vi "In Series_.vi"(7 "Tolerance (%)":dbl, 8 "error in (no error)":errorcluster, 9 "Number of Bands":T1=4 min=3 max=6 step=1, 10 "Resistance Digits":T2, 11 "E-Series Data":T5) -> (0 "error out":errorcluster, 3 "In Series?":T4)   [LabVIEW 2018]
doc: "Determines the E-Series membership of a resistor based on its number of bands, tolerance, and significant digits.\n\nThe VI receives the <b>E-Series Data</b>, <b>Tolerance (%)</b>, <b>Number of Bands</b>, and <b>Resistance Digits</b>. It uses <b>Build Resistor Cipher.vi</b> to construct the resistance value represented by the selected digits.\n\nBased on the number of bands and the resistor tolerance, the VI evaluates the applicable E-Series values and determines which series contain the resistance value.\n\nThe result is returned through <b>In Series?</b>, a cluster of Boolean indicators corresponding to E3, E6, E12, E24, E48, E96, and E192.\n\nThe VI propagates errors through its <b>error in</b> and <b>error out</b> terminals."
uses:
  E-Series Reader/Series Data--cluster.ctl
  In series--cluster.ctl
  Resistance Digits--cluster.ctl
  Ddigit--enum.ctl
  Number of Bands--number.ctl
  Resistance Value/Resistance Value.lvlib
  E-Series Reader/E-Series Reader.lvlib
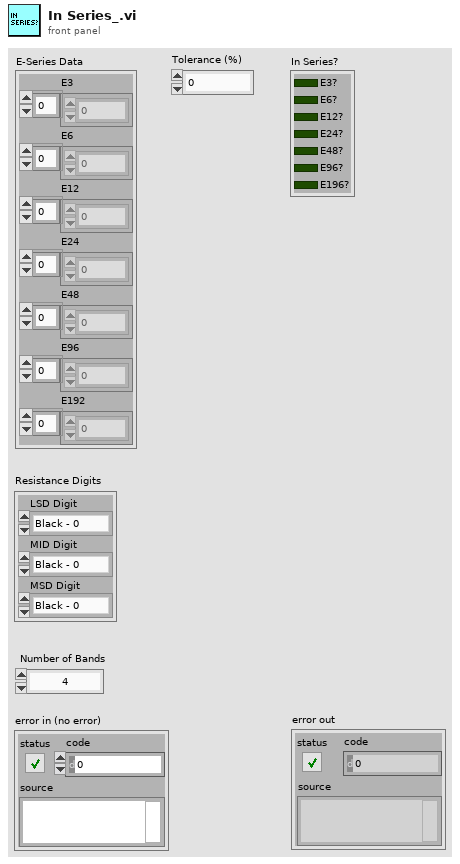
[diagram p1: front panel]
types:
  T1 = typedef "Number of Bands--number.ctl" = u8
  T2 = typedef "Resistance Digits--cluster.ctl" = cluster{"LSD Digit":T3, "MID Digit":T3, "MSD Digit":T3}
  T3 = typedef "Ddigit--enum.ctl" = enum16{"Black - 0", "Brown - 1", "Red - 2", "Orange - 3", "Yellow - 4", "Green - 5", "Blue - 6", "Violet - 7", "Grey - 8", "White - 9"}
  T4 = typedef "In series--cluster.ctl" = cluster{"E3?":bool, "E6?":bool, "E12?":bool, "E24?":bool, "E48?":bool, "E96?":bool, "E196?":bool}
  T5 = typedef "E-Series Reader.lvlib/Series Data--cluster.ctl" = cluster{"E3":u16[], "E6":u16[], "E12":u16[], "E24":u16[], "E48":u16[], "E96":u16[], "E192":u16[]}
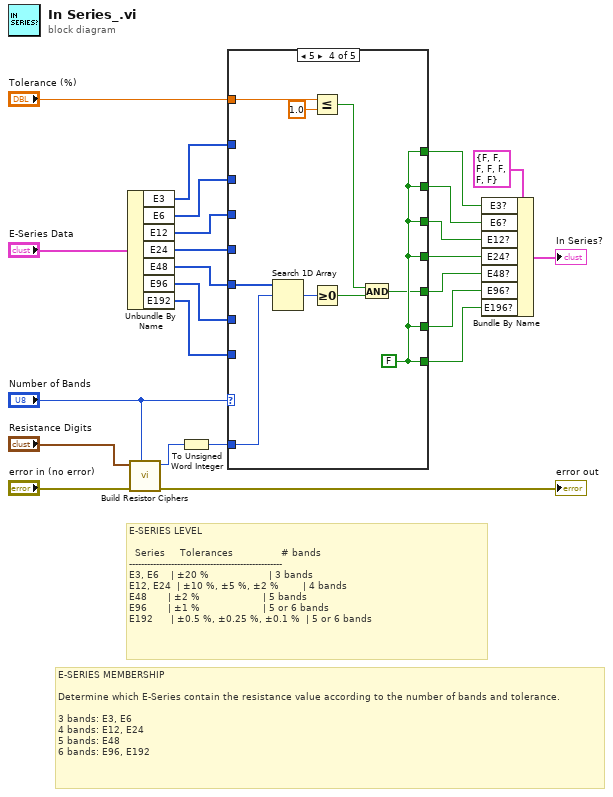
[diagram p0: block diagram]
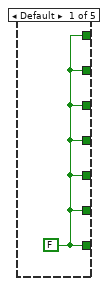
[diagram p2: hidden frame]
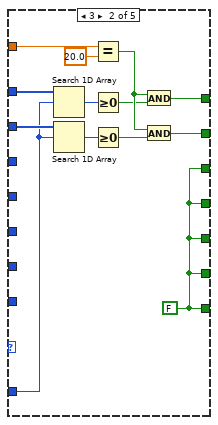
[diagram p3: hidden frame]
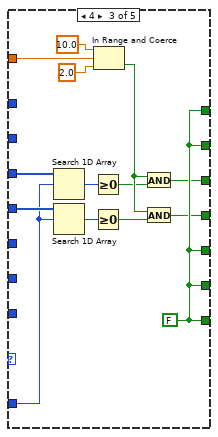
[diagram p4: hidden frame]
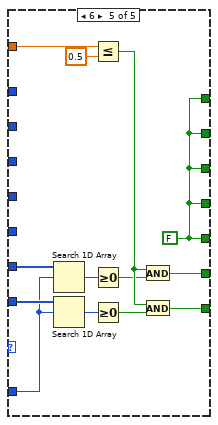
[diagram p5: hidden frame]
diagram:
  # "E-SERIES MEMBERSHIP\n\nDetermine which E-Series contain the resistance value according to the number of bands and tolerance.\n\n3 bands: E3, E6\n4 bands: E12, E24\n5 bands: E48\n6 bands: E96, E192"
  # "E-SERIES LEVEL\n\n  Series     Tolerances                # bands\n---------------------------------------------------\nE3, E6    | ±20 %                    | 3 bands\nE12, E24  | ±10 %, ±5 %, ±2 %        | 4 bands\nE48       | ±2 %                     | 5 bands\nE96       | ±1 %                     | 5 or 6 bands\nE192      | ±0.5 %, ±0.25 %, ±0.1 %  | 5 or 6 bands"
  n1 = Unbundle By Name("E-Series Data") -> ("E3"=w8:u16[], "E6"=w7:u16[], "E12"=w5:u16[], "E24"=w4:u16[], "E48"=w3:u16[], "E96"=w2:u16[], "E192"=w1:u16[])
  n2 = call "Build Resistor Ciphers.vi"("Number of Bands"="Number of Bands", "error in (no error)"="error in (no error)", "Resistance Digits"="Resistance Digits") -> ("error out"=→"error out":errorcluster, "Nominal Value"=w22:i32)  [unwired: 6 in, 1 out]
  n3 = To Unsigned Word Integer(number=w22) -> (unsigned 16bit integer=w6:u16)
  n4 = case shown="5" "Number of Bands" {
    tunnel: [w25 w34 w52 w61 w74] -> w18
    tunnel: [w25 w33 w52 w61 w74] -> w14
    tunnel: [w25 w38 w47 w61 w74] -> w13
    tunnel: [w25 w38 w46 w61 w74] -> w12
    tunnel: [w25 w38 w52 w61 w70] -> w16
    tunnel: [w25 w38 w52 w61 w69] -> w17
    tunnel: [w25 w38 w52 w58 w74] -> w15
    tunnel: "Tolerance (%)" -> [_ w37 w49 w60 w72]
    tunnel: w8 -> [_ w28 _ _ _]
    tunnel: w7 -> [_ w27 _ _ _]
    tunnel: w6 -> [_ w26 w39 w53 w62]
    tunnel: w5 -> [_ _ w41 _ _]
    tunnel: w4 -> [_ _ w40 _ _]
    tunnel: w3 -> [_ _ _ w54 _]
    tunnel: w2 -> [_ _ _ _ w64]
    tunnel: w1 -> [_ _ _ _ w63]
    frame Default {
      w25 = FALSE
    }
    frame 3 {
      w38 = FALSE
      n5 = Search 1D Array(1D array=w28, element=w26) -> (index of element=w31:i32)  [unwired: 1 in]
      n6 = Search 1D Array(1D array=w27, element=w26) -> (index of element=w32:i32)  [unwired: 1 in]
      n7 = Equal?(x=w37, y=20.0) -> (x = y?=w35:bool)
      n8 = Greater Or Equal To 0?(x=w31) -> (x >= 0?=w30:bool)
      n9 = Greater Or Equal To 0?(x=w32) -> (x >= 0?=w29:bool)
      n10 = And(x=w35, y=w30) -> (x .and. y?=w34:bool)
      n11 = And(x=w35, y=w29) -> (x .and. y?=w33:bool)
    }
    frame 4 {
      w52 = FALSE
      n12 = Search 1D Array(1D array=w41, element=w39) -> (index of element=w44:i32)  [unwired: 1 in]
      n13 = Search 1D Array(1D array=w40, element=w39) -> (index of element=w45:i32)  [unwired: 1 in]
      n14 = Greater Or Equal To 0?(x=w44) -> (x >= 0?=w43:bool)
      n15 = Greater Or Equal To 0?(x=w45) -> (x >= 0?=w42:bool)
      n16 = In Range and Coerce(upper limit=10.0 ("x"), x=w49, lower limit=2.0) -> (In Range?=w48:bool)  [unwired: 1 out]
      n17 = And(x=w48, y=w43) -> (x .and. y?=w47:bool)
      n18 = And(x=w48, y=w42) -> (x .and. y?=w46:bool)
    }
    frame 5 {
      w61 = FALSE
      n19 = Search 1D Array(1D array=w54, element=w53) -> (index of element=w56:i32)  [unwired: 1 in]
      n20 = Less Or Equal?(x=w60, y=1.0) -> (x <= y?=w57:bool)
      n21 = Greater Or Equal To 0?(x=w56) -> (x >= 0?=w55:bool)
      n22 = And(x=w57, y=w55) -> (x .and. y?=w58:bool)
    }
    frame 6 {
      w74 = FALSE
      n23 = Search 1D Array(1D array=w64, element=w62) -> (index of element=w68:i32)  [unwired: 1 in]
      n24 = Search 1D Array(1D array=w63, element=w62) -> (index of element=w67:i32)  [unwired: 1 in]
      n25 = Less Or Equal?(x=w72, y=0.5) -> (x <= y?=w71:bool)
      n26 = Greater Or Equal To 0?(x=w68) -> (x >= 0?=w65:bool)
      n27 = Greater Or Equal To 0?(x=w67) -> (x >= 0?=w66:bool)
      n28 = And(x=w71, y=w65) -> (x .and. y?=w70:bool)
      n29 = And(x=w71, y=w66) -> (x .and. y?=w69:bool)
    }
  }
  n30 = Bundle By Name(cluster=T4 {"E3?"=FALSE, "E6?"=FALSE, "E12?"=FALSE, "E24?"=FALSE, "E48?"=FALSE, "E96?"=FALSE, "E196?"=FALSE} ("In Series?"), "E3?"=w18, "E6?"=w14, "E12?"=w13, "E24?"=w12, "E48?"=w15, "E96?"=w16, "E196?"=w17) -> (→"In Series?":T4)
